vi "change_ConfigDialog.vi"(6 "CAl":T6, 8 "tag and parent tag":cluster{"tag":string, "parent tag":string}, 9 "value":string[](array[string]), 10 "Enum":T7=enum."CName", 11 "configtable":T3 {"CHS"."display" format="%b"}) -> (2 "all device out":T3 {"CHS"."display" format="%b"})   [LabVIEW 2011]
uses:
  contable.ctl
  CHS.ctl
  singlechtype.ctl
  config table enum.ctl
  signal type.ctl
  gain.ctl
panel:
  in  "Gain":T1
  in  "type":T2
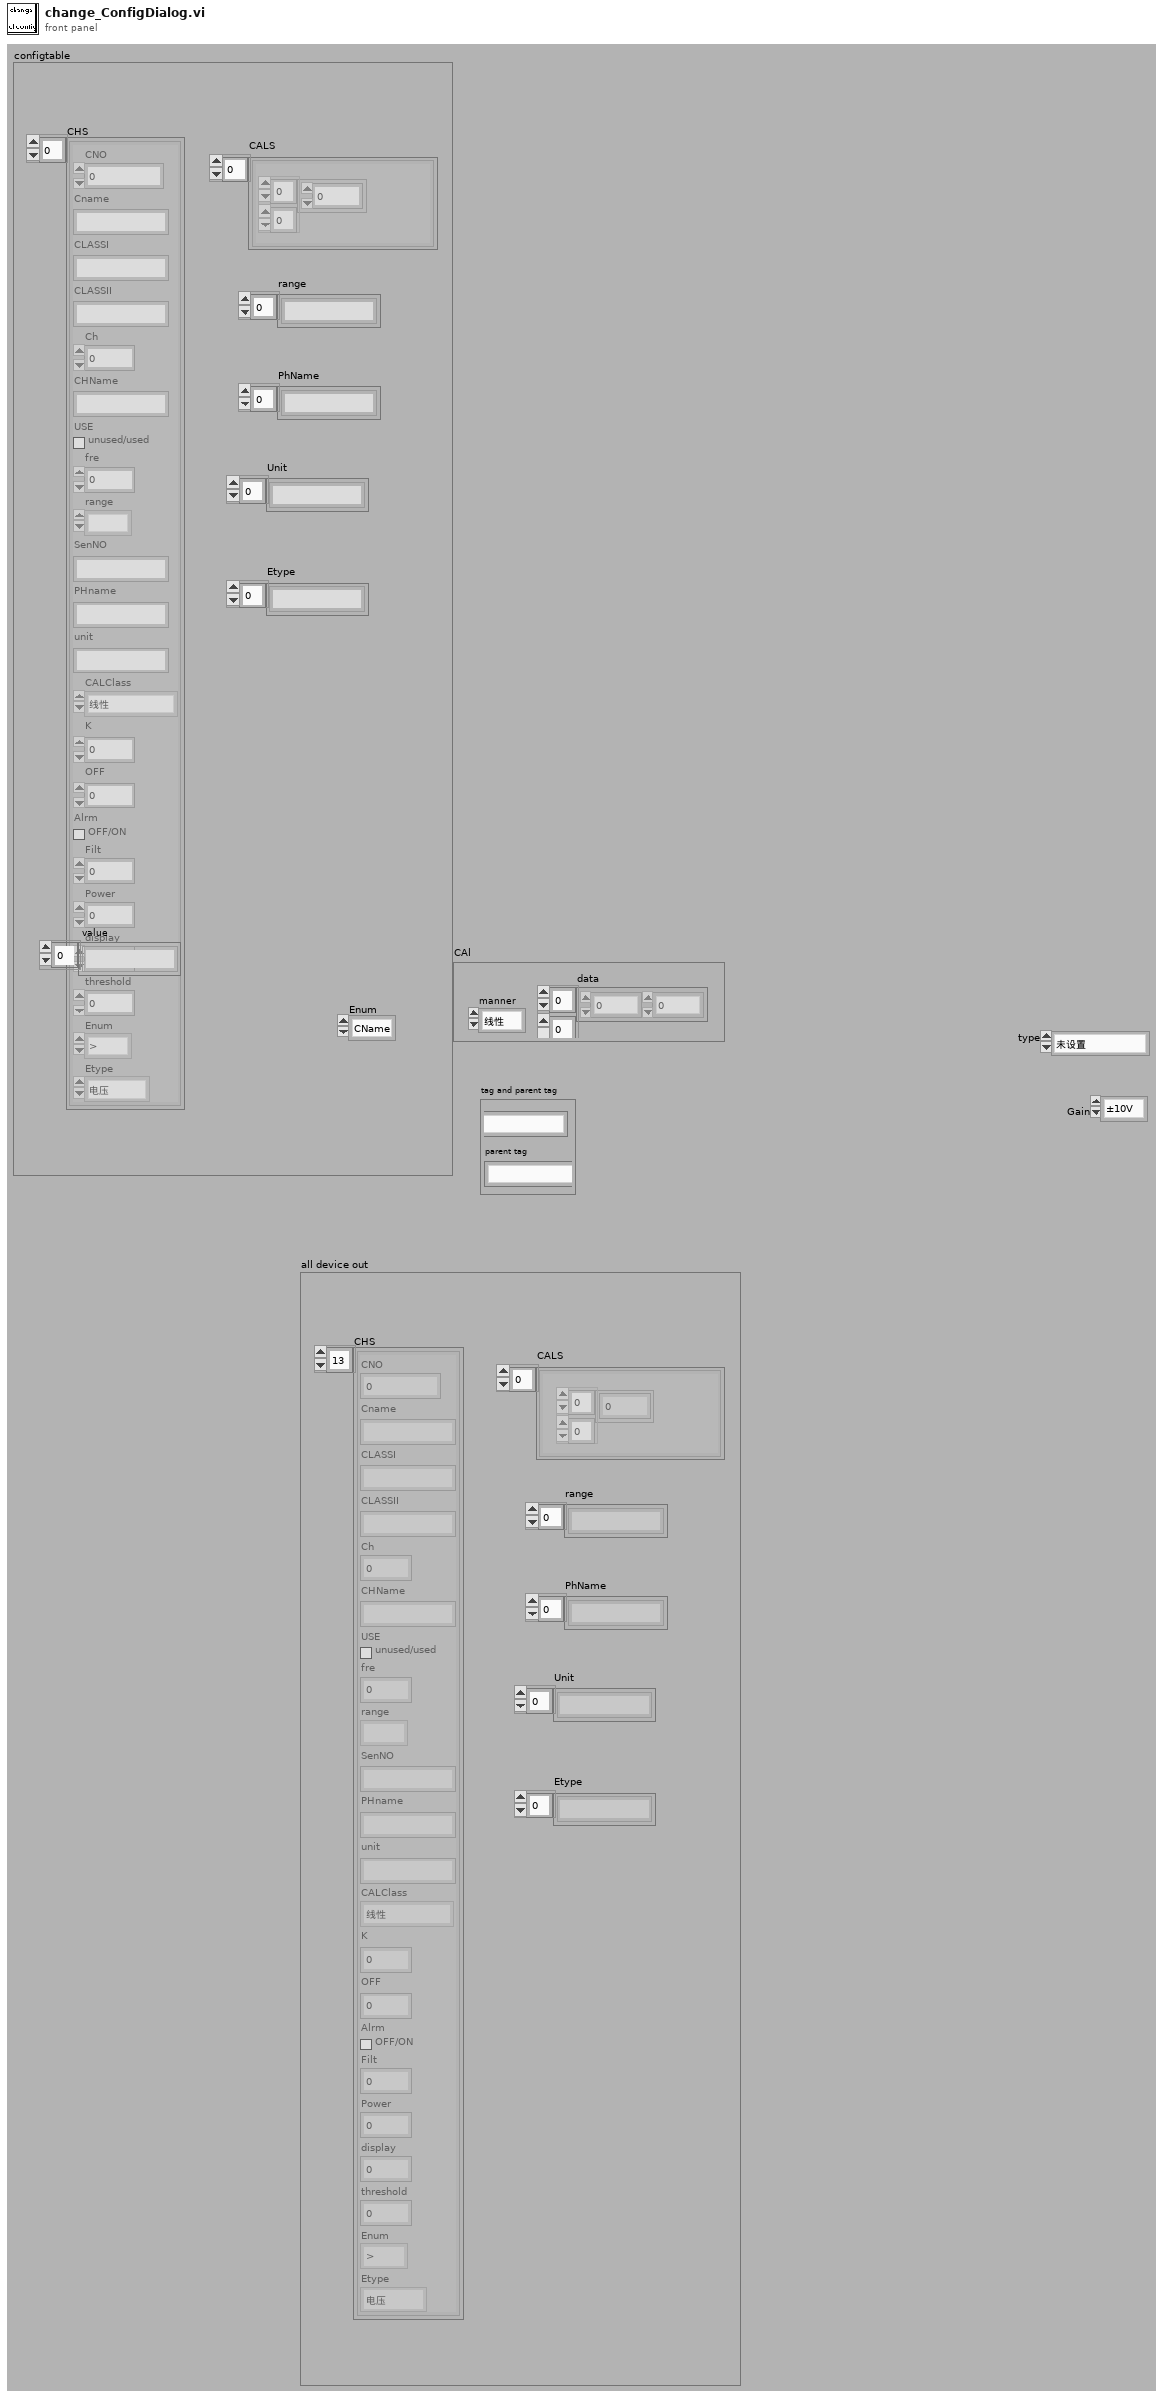
[diagram p1: front panel]
types:
  T1 = typedef "gain.ctl" = enum16{"±10V", "±5V", "±2.5V", "±1V", "±500mV", "±100mV", "10V", "5V", "2.5V", "1V", "500mV", "100mV"}
  T2 = typedef "signal type.ctl" = enum16{"未设置", "volet", "current", "vibration", "electric charge ", "resistance "}
  T3 = typedef "contable.ctl" = cluster{"CHS":T4, "CALS":cluster{"Array":dbl[][]}[], "range":string[], "PhName":string[], "Unit":string[], "Etype":string[]}
  T4 = typedef "CHS.ctl" = T5[]
  T5 = typedef "singlechtype.ctl" = cluster{"CNO":u8, "Cname":string, "CLASSI":string, "CLASSII":string, "Ch":u8, "CHName":string, "USE":bool, "fre":dbl, "range":enum16{""}, "SenNO":string, "PHname":string, "unit":string, "CALClass":enum8{"线性", "查表", "公式"}, "K":dbl, "OFF":dbl, "Alrm":bool, "Filt":dbl, "Power":u8, "display":u8, "threshold ":dbl, "Enum":enum16{">", ">=", "<", "<=", "<>(在范围内）", "><（在范围外）"}, "Etype":enum16{"电压", "电流", "电阻", "热电偶K", "热电偶T"}}
  T6 = cluster{"manner":enum16{"线性", "查表"}, "data":dbl[][]}
  T7 = typedef "config table enum.ctl" = enum16{"CNO.", "CName", "CLASSI", "CLASSII", "ch", "Chname", "USE", "fre", "range", "senNO", "PHname", "unit", "CALclass", "K", "OFF", "Alrm", "filt", "Power", "display", "threshold", "compare", "Etype"}
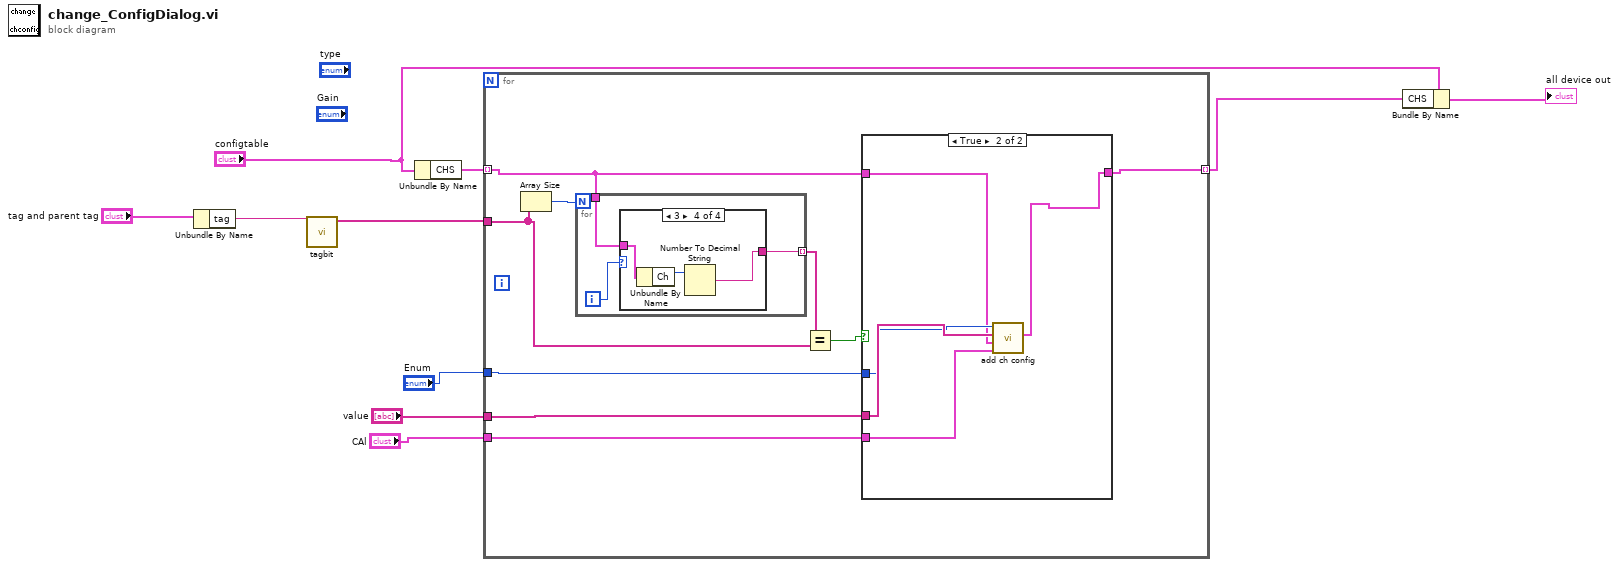
[diagram p0: block diagram]
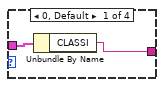
[diagram p2: hidden frame]
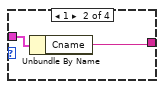
[diagram p3: hidden frame]
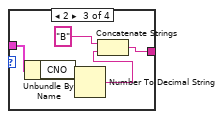
[diagram p4: hidden frame]
diagram:
  n1 = Unbundle By Name("tag and parent tag") -> ("tag"=w5:string)
  n2 = call "tagbit.vi"("tag"=w5) -> ("tag cell"=w4:string[])  [unwired: 8 in]
  n3 = Unbundle By Name("configtable") -> ("CHS"=w2:T4)
  n4 = for {
    tunnel: "Enum" -> [w15]
    tunnel: "value" -> [w19]
    tunnel: "CAl" -> [w18]
    tunnel: w4 -> [w12]
    tunnel: w2 -> [w16] mode=indexing
    tunnel: [w17] -> w3 mode=indexing
    n5 = Array Size(array=w12) -> (size(s)=w14:i32)
    n6 = for {
      N: w14 -> [_]
      tunnel: w16 -> [w22]
      tunnel: [w21] -> w13 mode=indexing
      i -> [w20]
      n7 = case shown="3" w20 {
        tunnel: [w24 w25 w29 w32] -> w21
        tunnel: w22 -> [w23 w26 w31 w34]
        frame 0, Default {
          n8 = Unbundle By Name(w23) -> ("CLASSI"=w24:string)
        }
        frame 1 {
          n9 = Unbundle By Name(w26) -> ("Cname"=w25:string)
        }
        frame 2 {
          n10 = Unbundle By Name(w31) -> ("CNO"=w30:u8)
          n11 = Number To Decimal String(number=w30) -> (decimal integer string=w27:string)  [unwired: 1 in]
          n12 = Concatenate Strings("B", w27) -> (w29:string)
        }
        frame 3 {
          n13 = Unbundle By Name(w34) -> ("Ch"=w33:u8)
          n14 = Number To Decimal String(number=w33) -> (decimal integer string=w32:string)  [unwired: 1 in]
        }
      }
    }
    n15 = Equal?(x=w13, y=w12) -> (x = y?=w11:bool)
    n16 = case shown="True" w11 {
      tunnel: w15 -> [_ w38]
      tunnel: w19 -> [_ w39]
      tunnel: w18 -> [_ w40]
      tunnel: w16 -> [w35 w36]
      tunnel: [w35 w37] -> w17
      frame False {
      }
      frame True {
        n17 = call "add ch config.vi"("CAl"=w40, "device chanel"=w36, "value"=w39, "Enum"=w38) -> ("device chanel out"=w37:T5)  [unwired: 1 in, 6 out]
      }
    }
  }
  n18 = Bundle By Name(cluster="configtable", "CHS"=w3) -> (→"all device out":T3)
